vi "Get Entry.vi"(10 "Section":string, 11 "EDS in":refnum<class "EDS.lvclass">) -> (2 "Object Entry":refnum<class "OD Section.lvclass">, 3 "EDS out":refnum<class "EDS.lvclass">)   [LabVIEW 2024, in "EDS.lvlib" / "EDS.lvclass"]
uses:
  EDS.lvclass
  EDS.lvclass/EDS.ctl
  Object Dictionary/Object Dictionary.lvclass
  OD Section/OD Section.lvclass
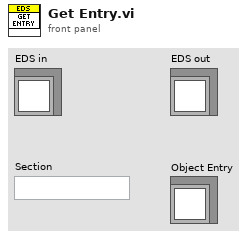
[diagram p1: front panel]
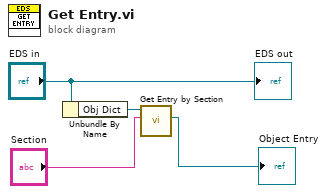
[diagram p0: block diagram]
diagram:
  n1 = Unbundle By Name("EDS in") -> ("Obj Dict"=w4:refnum<class "Object Dictionary.lvclass">)
  n2 = call "Get Entry by Section.vi"("Section"="Section", "Object Dictionary in"=w4) -> ("Object Entry out"=→"Object Entry":refnum<class "OD Section.lvclass">)  [unwired: 8 in, 1 out]
  "EDS out" <- "EDS in"
